vi "Initialize.vi"(7 "not in use":string="ActualValue.ch%d.AV", 8 "error in":errorcluster, 9 "Number of Channels":u32=1, 10 "Instance Name":string, 11 "Power Actual Value in":refnum<class "Power Actual Value.lvclass">) -> (0 "error out":errorcluster, 3 "Power Actual Value out":refnum<class "Power Actual Value.lvclass">)   [LabVIEW 2023, in "Power Actual Value.lvclass"]
uses:
  Power Actual Value.lvclass
  Parents/Actual Value/Actual Value.lvclass
  Power Actual Value.lvclass/Power Actual Value.ctl
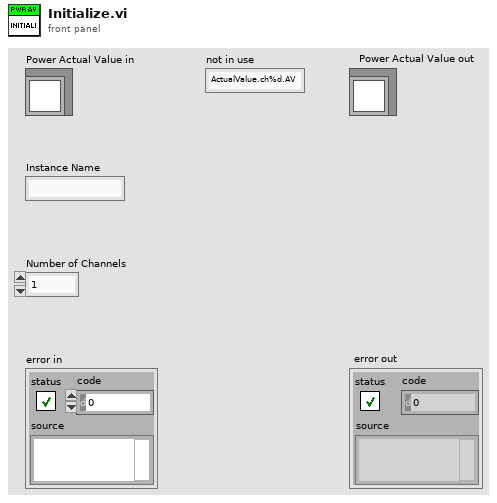
[diagram p1: front panel]
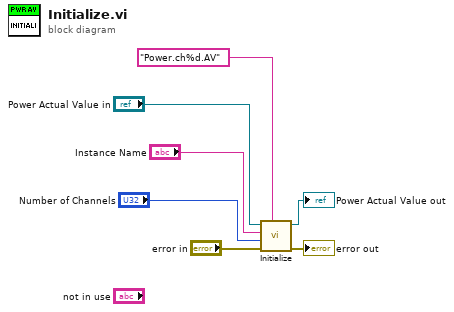
[diagram p0: block diagram]
diagram:
  n1 = call-parent "Initialize.vi"("ChannelName"="Power.ch%d.AV", "error in"="error in", "Number of Channels"="Number of Channels", "Instance Name"="Instance Name", "Actual Value in"="Power Actual Value in") -> ("error out"=→"error out":errorcluster, "Actual Value out"=→"Power Actual Value out":refnum<class "Power Actual Value.lvclass">)  [unwired: 5 in]
